vi "子界面-查看某框和报告生成.vi"(0 "框号":dbl format="%#_13g", 1 "框组":T4(array[cluster]), 2 "反射图":T1(plugin-control), 4 "标注图":T1(plugin-control)) -> ()   [LabVIEW 2018]
uses:
  <vilib>/vision/NI_Vision_Development_Module.lvlib
panel:
  in  "数据库UDL路径":path
  in  "写入数据库":bool
  out "ROI位置Y":i32
  out "ROI位置X":i32
  out "反射图ROI对应区域灰度表":u32[](graph)
  out "报告生成路径":path
  out "?":T1(plugin-control)
  out "Threshold Image":T1(plugin-control)
  in  "格式字符串 2":string="%f"
  in  "分隔符（'\\'代码显示）":string="\t"
  out "分层测量结果":dbl[][](array[numeric]) format="%.2f"
  out "分层类检测结果":string[][](table)
  out "Threshold Image":T1(plugin-control)
  out "Threshold Image":T1(plugin-control)
  out "缺陷分类的临界值":sgl
  out "反射图ROI的最大灰度值":sgl
  in  "返回 2":bool
  in  "报告生成":bool
  in  "反射法图像-面积阈值设置":T3(array[cluster]) {"Measurement Parameter" items=["Area"]; "下限" min=0 step=1; "上限" min=0 step=1}
  in  "穿透法图像-灰度阈值设置":cluster{"下限":dbl, "下限":dbl}(slide)={"下限"=0.0, "下限"=65.10638427734375} scale=0.0..255.0
  in  "保存结果":bool
  in  "部位":string
  in  "Color":u32[](array[colorbox])=[3381759, 16776770, 16777225, 6618880]
  in  "Overlay Type":u16[](array[ring])=[2, 1, 3, 0] items=["Rectangle", "Numbers", "Points", "Lines"]
  in  "Tab Control":T5
  out "穿透ROI":T1(plugin-control)
  out "Threshold Image":T1(plugin-control)
  out "?":T1(plugin-control)
  out "?":T1(plugin-control)
  out "Threshold Image":T1(plugin-control)
  out "Threshold Image":T1(plugin-control)
  out "弥散测量结果":dbl[][](array[numeric]) format="%.2f"
  in  "产品序号":string
  in  "测试人":string
  in  "分隔符（'\\'代码显示）":string="\t"
  in  "格式字符串":string="%f"
  out "弥散类检测结果":string[][](table)
  out "?":string
  out "面积 (pixels)":i32
  # "所选区域信息"
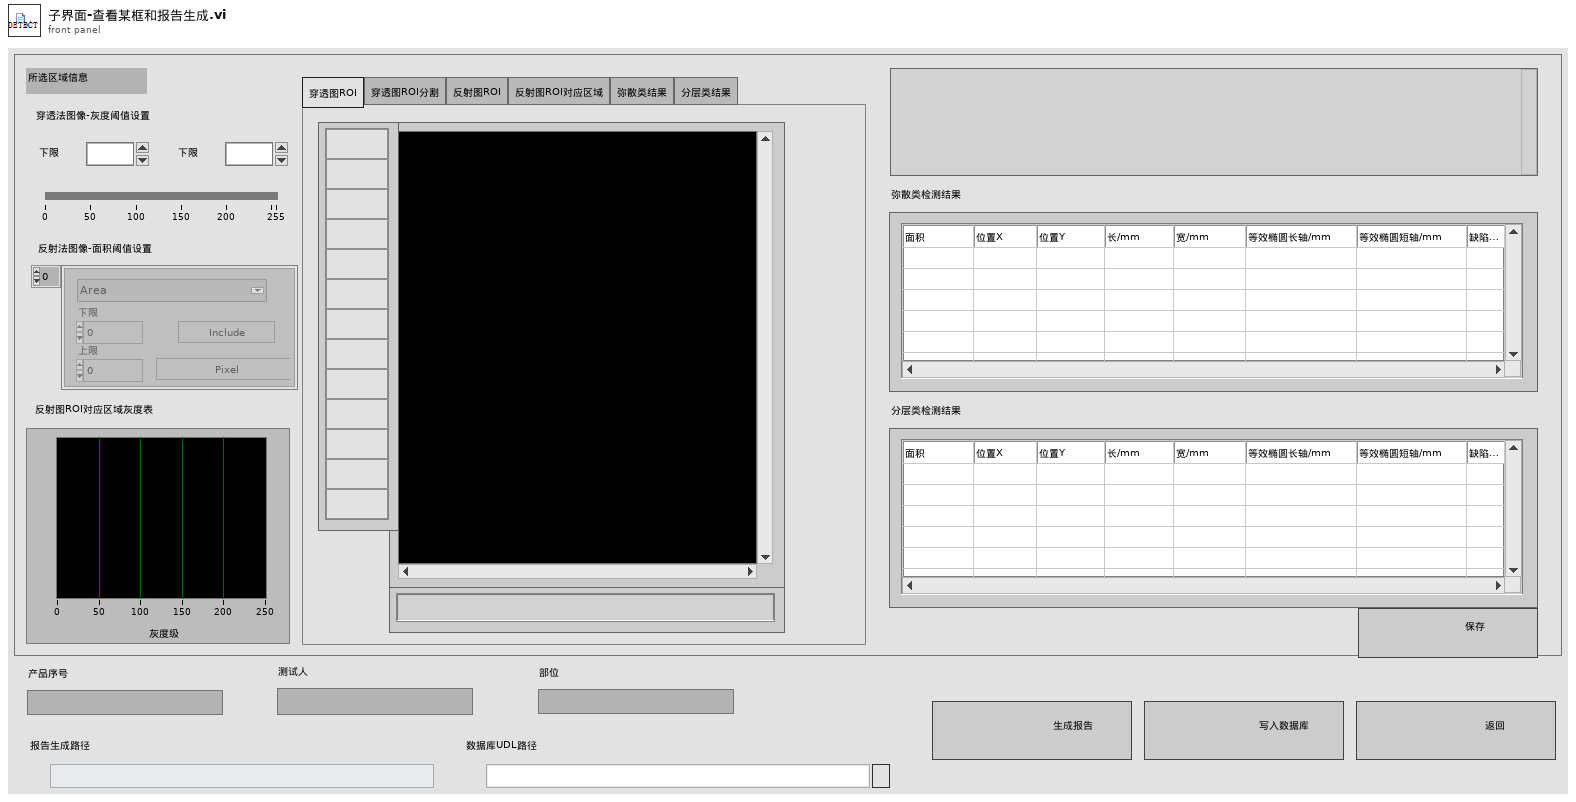
[diagram p1: front panel]
types:
  T1 = typedef "IMAQ Image.ctl" = refnum<image>
  T2 = typedef "Particle Parameters" = i32
  T3 = cluster{"Measurement Parameter":T2, "下限":i32, "上限":i32, "Range":bool, "Measurement Type":bool}[]
  T4 = cluster{"Global Rectangle":i32[], "Contours":cluster{"Contour Type":u32, "ROI Type":u32, "Points":i32[]}[]}[]
  T5 = typedef "控件 1.ctl" = enum32{"穿透图ROI", "穿透图ROI分割", "反射图ROI", "反射图ROI对应区域", "弥散类结果", "分层类结果"}
  T6 = typedef "Image Type" = u32
  T7 = cluster{"Global Rectangle":i32[], "Contours":cluster{"Contour Type":u32, "ROI Type":u32, "Points":i32[]}[]}
  T8 = cluster{"Pixel Measurements":T2[], "Overlay Type":u16[], "Color":u32[], "反射法图像-面积阈值设置":cluster{"Measurement Parameter":T2, "下限":i32, "上限":i32, "Range":bool, "Measurement Type":bool}[], "穿透法图像-灰度阈值设置":cluster{"下限":dbl, "下限":dbl}}
  T9 = cluster{"histogram":u32[], "Minimal Value":sgl, "Maximal Value":sgl, "Starting Value":sgl, "Interval Width":sgl, "Mean Value":sgl, "Standard  Variation":sgl, "Area (pixels)":i32}
  T10 = cluster{"Desired Font (Application)":enum16{"User-specified Font", "Application Font", "System Font", "Dialog Font"}, "[User-specified Font]":cluster{"Font Name":string, "Size":i16, "Strikeout?":bool, "Italic?":bool, "Underline?":bool, "Outline?":bool, "Shadow?":bool, "Bold?":bool, "Rotation Angle":dbl}, "Horizontal Alignment":i16, "Vertical Alignment":i16}
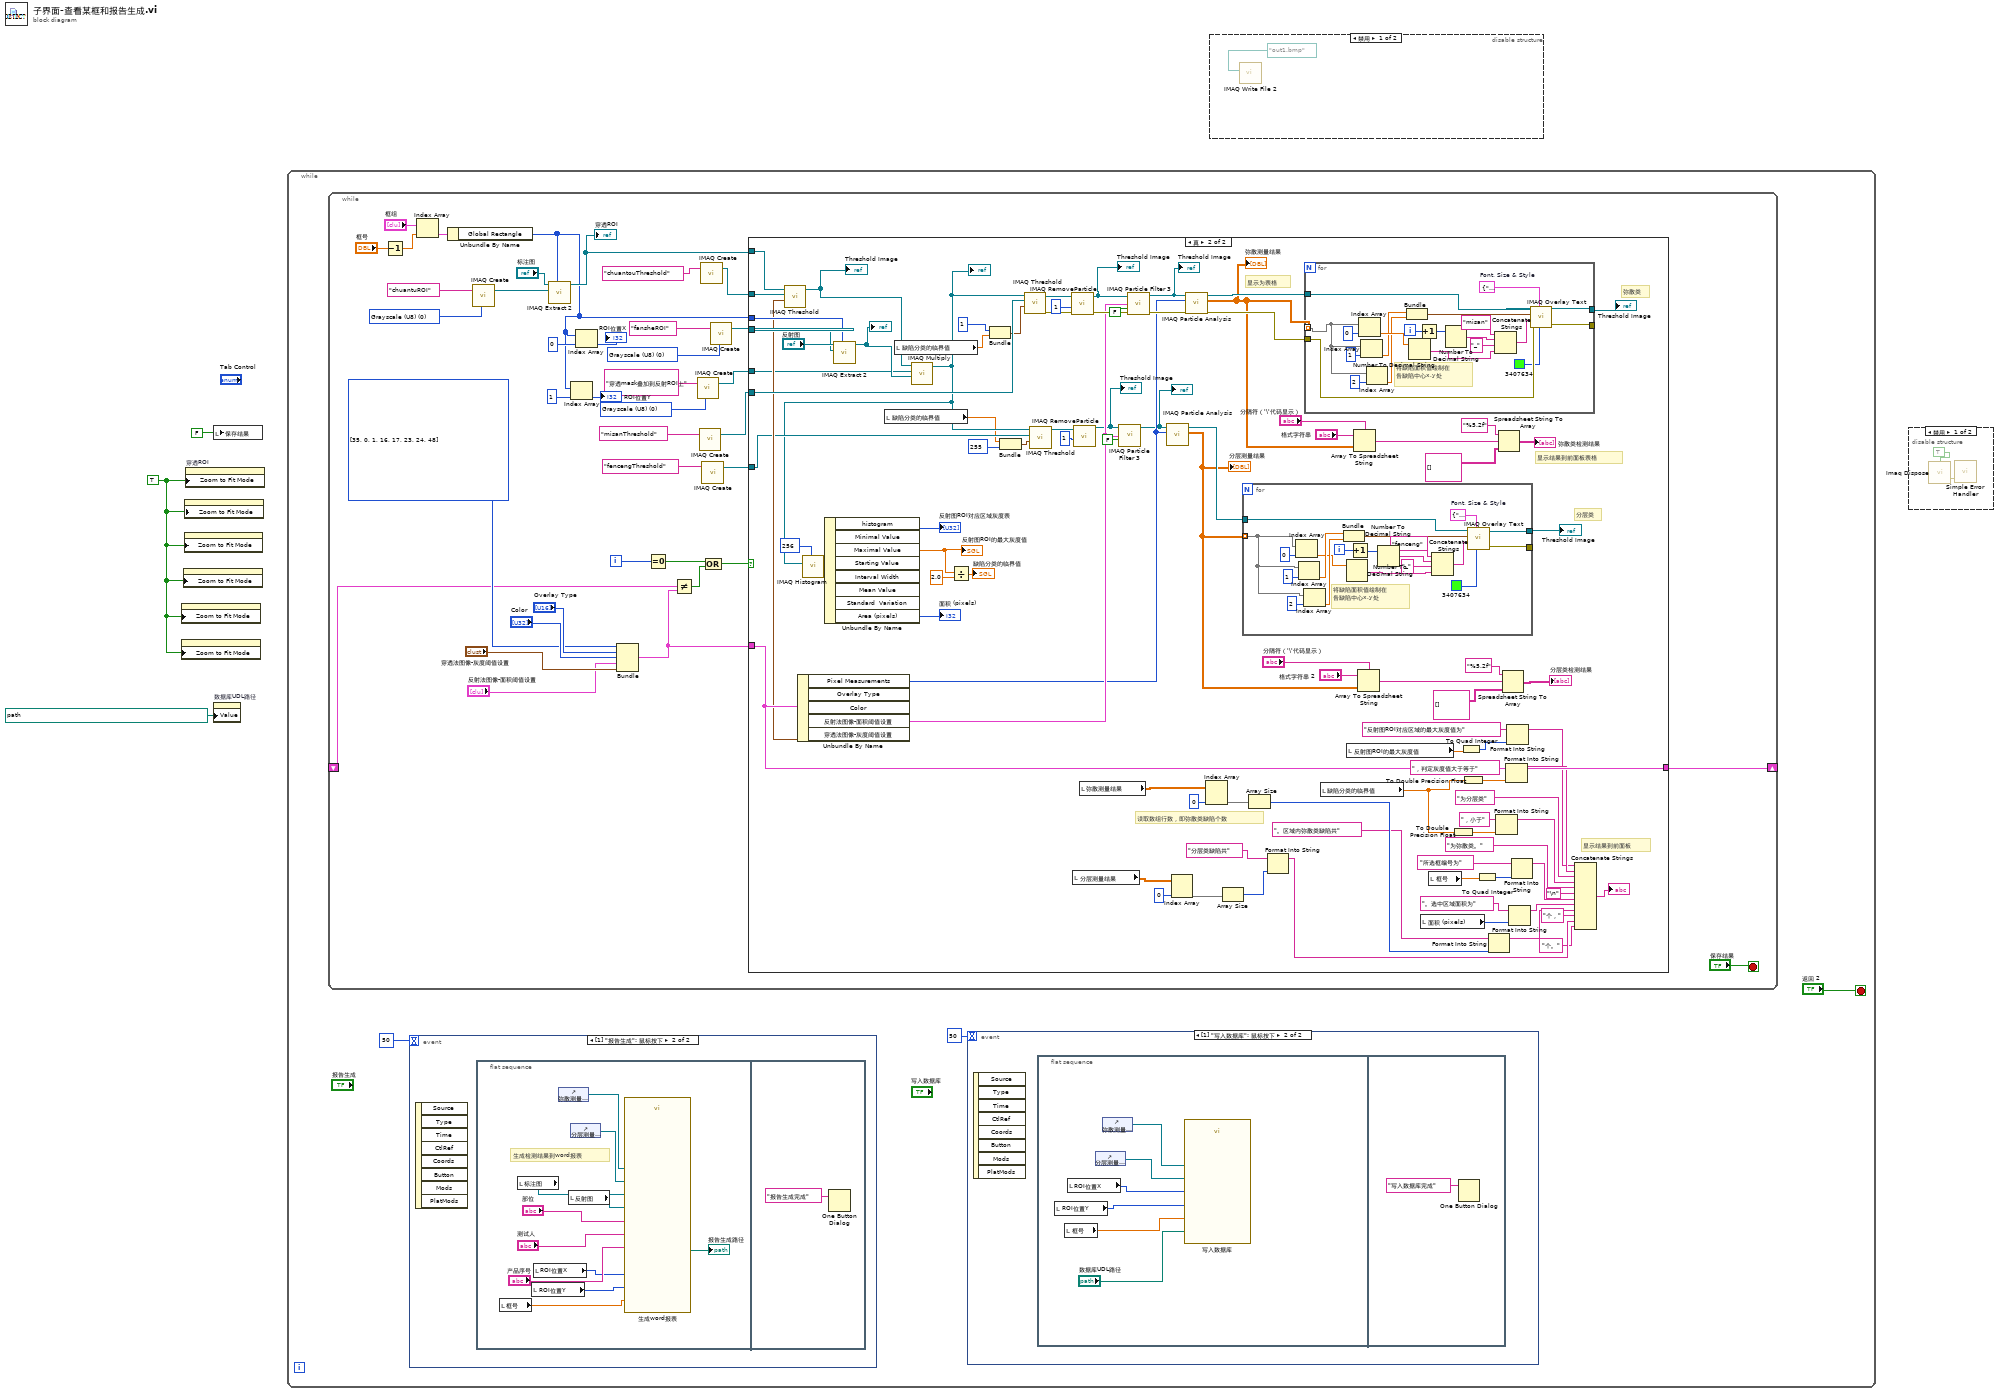
[diagram p0: block diagram]
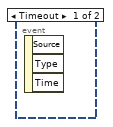
[diagram p3: hidden frame]
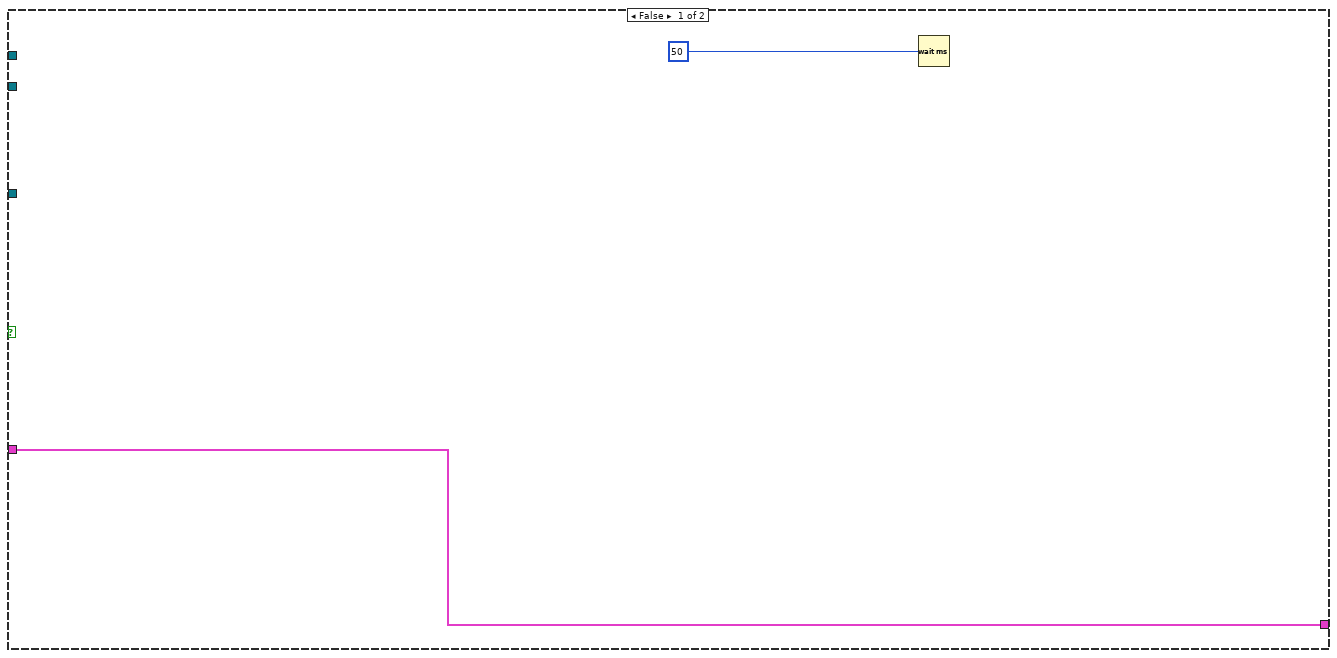
[diagram p4: hidden frame]
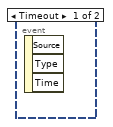
[diagram p5: hidden frame]
diagram:
  w2 = TRUE ("Zoom to Fit Mode")
  n1 = property class="ImageControl"("Zoom to Fit Mode"=w2) -> ()  [unwired: 2 in, 2 out]
  n2 = property class="ImageControl"("Zoom to Fit Mode"=w2) -> ()  [unwired: 2 in, 2 out]
  n3 = property class="ImageControl"("Zoom to Fit Mode"=w2) -> ()  [unwired: 2 in, 2 out]
  n4 = property class="ImageControl"("Zoom to Fit Mode"=w2) -> ()  [unwired: 2 in, 2 out]
  n5 = property class="ImageControl"("Zoom to Fit Mode"=w2) -> ()  [unwired: 2 in, 2 out]
  n6 = property on="穿透ROI" class="ImageControl"("Zoom to Fit Mode"=w2) -> ()  [unwired: 2 in, 2 out]
  n7 = local write "保存结果"(FALSE) -> ()
  n8 = property on="数据库UDL路径" class="Path"("Value"=path "E:/MyGithub/MyLabVIEW/晨光项目/代码/test.udl" ("数据库UDL路径")) -> ()  [unwired: 2 in, 2 out]
  n9 = while {
    stop <- "返回 2" stop-if-true
    n10 = while {
      shift-right: [w44] -> _
      shift-left: _ -> [w43]
      i -> [w48]
      stop <- "保存结果" stop-if-true
      w23 = T6 0 items=["Grayscale (U8)", "Grayscale (I16)", "Grayscale (SGL)", "Complex (CSG)", "RGB (U32)", "HSL (U32)", "RGB (U64)", "Grayscale (U16)"] ("Image Type")
      w29 = T6 0 items=["Grayscale (U8)", "Grayscale (I16)", "Grayscale (SGL)", "Complex (CSG)", "RGB (U32)", "HSL (U32)", "RGB (U64)", "Grayscale (U16)"] ("Image Type")
      w35 = T6 0 items=["Grayscale (U8)", "Grayscale (I16)", "Grayscale (SGL)", "Complex (CSG)", "RGB (U32)", "HSL (U32)", "RGB (U64)", "Grayscale (U16)"] ("Image Type")
      w50 = T2[] [35, 0, 1, 16, 17, 23, 24, 48] items=["Center of Mass X", "Center of Mass Y", "First Pixel X", "First Pixel Y", "Bounding Rect Left", "Bounding Rect Top", "Bounding Rect Right", "Bounding Rect Bottom", "Max Feret Diameter Start X", "Max Feret Diameter Start Y", "Max Feret Diameter End X", "Max Feret Diameter End Y", "Max Horiz. Segment Length Left", "Max Horiz. Segment Length Right", "Max Horiz. Segment Length Row", "-", "Bounding Rect Width", "Bounding Rect Height", "Bounding Rect Diagonal", "Perimeter", "Convex Hull Perimeter", "Holes' Perimeter", "Max Feret Diameter", "Equivalent Ellipse Major Axis", "Equivalent Ellipse Minor Axis", "Equivalent Ellipse Minor Axis (Feret)", "Equivalent Rect Long Side", "Equivalent Rect Short Side", "Equivalent Rect Diagonal", "Equivalent Rect Short Side (Feret)", "Average Horiz. Segment Length", "Average Vert. Segment Length", "Hydraulic Radius", "Waddel Disk Diameter", "-", "Area", "Holes' Area", "Particle & Holes' Area", "Convex Hull Area", "Image Area", "-", "Number of Holes", "Number of Horiz. Segments", "Number of Vert. Segments", "-", "Orientation", "Max Feret Diameter Orientation", "-", "% Area/Image Area", "% Area/(Particle & Holes' Area)", "Ratio of Equivalent Ellipse Axes", "Ratio of Equivalent Rect Sides", "-", "Elongation Factor", "Compactness Factor", "Heywood Circularity Factor", "Type Factor", "-", "Sum X", "Sum Y", "Sum XX", "Sum XY", "Sum YY", "Sum XXX", "Sum XXY", "Sum XYY", "Sum YYY", "-", "Moment of Inertia XX", "Moment of Inertia XY", "Moment of Inertia YY", "Moment of Inertia XXX", "Moment of Inertia XXY", "Moment of Inertia XYY", "Moment of Inertia YYY", "Norm. Moment of Inertia XX", "Norm. Moment of Inertia XY", "Norm. Moment of Inertia YY", "Norm. Moment of Inertia XXX", "Norm. Moment of Inertia XXY", "Norm. Moment of Inertia XYY", "Norm. Moment of Inertia YYY", "Hu Moment 1", "Hu Moment 2", "Hu Moment 3", "Hu Moment 4", "Hu Moment 5", "Hu Moment 6", "Hu Moment 7"] ("Pixel Measurements")
      n11 = Decrement(x="框号") -> (x-1=w37:dbl)
      n12 = Index Array(array="框组", index=w37) -> (element=w39:T7)
      n13 = Unbundle By Name(w39) -> ("Global Rectangle"=w15:i32[])
      n14 = call "IMAQ Create"("Image Name"="chuantuROI", "Image Type"=w35) -> ("New Image"=w38:T1)  [unwired: 3 in, 1 out]
      n15 = call "IMAQ Extract 2"("Optional Rectangle"=w15, "Image Dst"=w38, "Image Src"="标注图") -> ("Image Dst Out"=w26:T1)  [unwired: 7 in, 1 out]
      "穿透ROI" <- w26
      n16 = Index Array(array=w15, index=1 ("索引")) -> (element=→"ROI位置Y":i32)
      n17 = Index Array(array=w15, index=0 ("索引")) -> (element=→"ROI位置X":i32)
      n18 = Bundle("Pixel Measurements"=w50, "Overlay Type"="Overlay Type", "Color"="Color", "反射法图像-面积阈值设置"="反射法图像-面积阈值设置", "穿透法图像-灰度阈值设置"="穿透法图像-灰度阈值设置") -> (w27:T8)  [unwired: 1 in]
      n19 = Equal To 0?(x=w48) -> (x = 0?=w47:bool)
      n20 = Not Equal?(x=w43, y=w27) -> (x != y?=w46:bool)
      n21 = call "IMAQ Create"("Image Name"="穿透mask叠加到反射ROI上", "Image Type"=w23) -> ("New Image"=w22:T1)  [unwired: 3 in, 1 out]
      n22 = call "IMAQ Create"("Image Name"="misanThreshold") -> ("New Image"=w21:T1)  [unwired: 4 in, 1 out]
      n23 = call "IMAQ Create"("Image Name"="chuantouThreshold") -> ("New Image"=w31:T1)  [unwired: 4 in, 1 out]
      n24 = call "IMAQ Create"("Image Name"="fencengThreshold") -> ("New Image"=w19:T1)  [unwired: 4 in, 1 out]
      n25 = Compound Arithmetic op=OR(w47, w46) -> (w45:bool)
      n26 = call "IMAQ Create"("Image Name"="fansheROI", "Image Type"=w29) -> ("New Image"=w28:T1)  [unwired: 3 in, 1 out]
      n27 = case shown="真" w45 {
        tunnel: w27 -> [w53 w116]
        tunnel: [w53 w116] -> w44
        tunnel: w31 -> [_ w124]
        tunnel: w26 -> [_ w114]
        tunnel: w28 -> [_ w122]
        tunnel: w15 -> [_ w121]
        tunnel: w21 -> [_ w120]
        tunnel: w22 -> [_ w111]
        tunnel: w19 -> [_ w83]
        frame False {
          n28 = Wait (ms)(milliseconds to wait=u32 50) -> ()  [unwired: 1 out]
        }
        frame True {
          # "分层类"
          # "弥散类"
          # "显示结果到前面板"
          # "读取数组行数，即弥散类缺陷个数"
          # "显示结果到前面板表格"
          # "显示为表格"
          n29 = Unbundle By Name(w116) -> ("Pixel Measurements"=w74:T2[], "反射法图像-面积阈值设置"=w76:T3, "穿透法图像-灰度阈值设置"=w115:cluster{"下限":dbl, "下限":dbl})  [unwired: 2 out]
          n30 = call "IMAQ Threshold"("Range"=w115, "Image Dst"=w124, "Image Src"=w114) -> ("Image Dst Out"=w113:T1)  [unwired: 3 in, 5 out]
          "Threshold Image" <- w113
          n31 = call "IMAQ Extract 2"("Optional Rectangle"=w121, "Image Dst"=w122, "Image Src"="反射图") -> ("Image Dst Out"=w112:T1)  [unwired: 7 in, 1 out]
          "?" <- w112
          n32 = local read "缺陷分类的临界值"() -> (w79:sgl)
          n33 = local read "缺陷分类的临界值"() -> (w90:sgl)
          n34 = call "IMAQ Multiply"("Image Src A"=w113, "Image Dst"=w111, "Image Src B"=w112) -> ("Image Dst Out"=w82:T1)  [unwired: 4 in, 1 out]
          "?" <- w82
          n35 = call "IMAQ Histogram"("Number of Classes"=256, "Image"=w82) -> ("Histogram Report"=w119:T9)  [unwired: 8 in, 1 out]
          n36 = Unbundle By Name(w119) -> ("histogram"=→"反射图ROI对应区域灰度表":u32[], "Maximal Value"=w107:sgl, "Area (pixels)"=→"面积 (pixels)":i32)  [unwired: 5 out]
          "反射图ROI的最大灰度值" <- w107
          n37 = Divide(x=w107, y=sgl 2.0) -> (x/y=→"缺陷分类的临界值":sgl)
          n38 = Bundle(1, "缺陷分类的临界值"=w90) -> (w89:cluster{i32, "缺陷分类的临界值":sgl})  [unwired: 1 in]
          n39 = Bundle("缺陷分类的临界值"=w79, 255) -> (w81:cluster{"缺陷分类的临界值":sgl, i32})  [unwired: 1 in]
          n40 = call "IMAQ Threshold"("Range"=w89, "Image Dst"=w120, "Image Src"=w82) -> ("error out"=w148:errorcluster, "Image Dst Out"=w125:T1)  [unwired: 3 in, 4 out]
          n41 = call "IMAQ Threshold"("Range"=w81, "Image Dst"=w83, "Image Src"=w82) -> ("Image Dst Out"=w78:T1)  [unwired: 3 in, 5 out]
          n42 = call "IMAQ RemoveParticle"("error in (no error)"=w148, "Number of Erosion"=1, "Image Src"=w125) -> ("error out"=w147:errorcluster, "Image Dst Out"=w87:T1)  [unwired: 7 in]
          "Threshold Image" <- w87
          n43 = local read "分层测量结果"() -> (w62:dbl[][])
          n44 = call "IMAQ RemoveParticle"("Number of Erosion"=1, "Image Src"=w78) -> ("Image Dst Out"=w57:T1)  [unwired: 8 in, 1 out]
          "Threshold Image" <- w57
          n45 = local read "弥散测量结果"() -> (w84:dbl[][])
          n46 = call "IMAQ Particle Filter 3"("Image Src"=w57, "Selection Values"=w76, "Keep/Remove Particles (F)"=FALSE) -> ("Image Dst Out"=w56:T1)  [unwired: 10 in, 2 out]
          "?" <- w56
          n47 = call "IMAQ Particle Filter 3"("Image Src"=w87, "Selection Values"=w76, "Keep/Remove Particles (F)"=FALSE, "error in (no error)"=w147) -> ("Image Dst Out"=w86:T1, "error out"=w146:errorcluster)  [unwired: 9 in, 1 out]
          "Threshold Image" <- w86
          n48 = call "IMAQ Particle Analysis"("Pixel Measurements"=w74, "Image"=w56) -> ("Particle Measurements (Pixels)"=w68:dbl[][], "Image Out (duplicate)"=w73:T1)  [unwired: 4 in, 4 out]
          "分层测量结果" <- w68
          n49 = Index Array(array=w62, index (col)=0 ("禁用的索引 (列)")) -> (element=w64:dbl[])  [unwired: 1 in]
          n50 = call "IMAQ Particle Analysis"("error in (no error)"=w146, "Pixel Measurements"=w74, "Image"=w86) -> ("error out"=w144:errorcluster, "Particle Measurements (Pixels)"=w126:dbl[][], "Image Out (duplicate)"=w145:T1)  [unwired: 3 in, 3 out]
          "弥散测量结果" <- w126
          n51 = Index Array(array=w84, index (col)=0 ("禁用的索引 (列)")) -> (element=w132:dbl[])  [unwired: 1 in]
          n52 = Array Size(array=w64) -> (size(s)=w60:i32)
          n53 = for {
            tunnel: [w170] -> _
            tunnel: [w169] -> w72
            tunnel: w73 -> [w156]
            tunnel: w68 -> [w154] mode=indexing
            i -> [w151]
            w167 = T10 {"Desired Font (Application)"=enum."Application Font", "[User-specified Font]"={"Font Name"="", "Size"=12, "Strikeout?"=FALSE, "Italic?"=FALSE, "Underline?"=FALSE, "Outline?"=FALSE, "Shadow?"=FALSE, "Bold?"=FALSE, "Rotation Angle"=0.0}, "Horizontal Alignment"=0, "Vertical Alignment"=0}  # Font, Size & Style
            # "将缺陷面积值绘制在\n各缺陷中心x,y处"
            n54 = Index Array(array=w154, index=0 ("索引")) -> (element=w153:dbl)
            n55 = Index Array(array=w154, index=1 ("索引")) -> (element=w164:dbl)
            n56 = Index Array(array=w154, index=2 ("索引")) -> (element=w162:dbl)
            n57 = Bundle("Numeric"=w164, "Numeric"=w162) -> (w155:cluster{"Numeric":dbl, "Numeric":dbl})  [unwired: 1 in]
            n58 = Number To Decimal String(number=w153) -> (decimal integer string=w159:string)  [unwired: 1 in]
            n59 = Increment(x=w151) -> (x+1=w152:i32)
            n60 = Number To Decimal String(number=w152) -> (decimal integer string=w161:string)  [unwired: 1 in]
            n61 = Concatenate Strings("fenceng" ("字符串"), w161, "_", w159) -> (w158:string)
            n62 = call "IMAQ Overlay Text"("Text Color (black)"=u32 3407634, "Font, Size & Style"=w167, "String"=w158, "Origin"=w155, "Image"=w156) -> ("error out"=w170:errorcluster, "Image Out"=w169:T1)  [unwired: 5 in]
          }
          "Threshold Image" <- w72
          n63 = Array Size(array=w132) -> (size(s)=w134:i32)
          n64 = Format Into String(initial string="分层类缺陷共" ("初始字符串"), w60) -> (resulting string=w59:string)  [unwired: 2 in, 1 out]
          n65 = for {
            tunnel: w144 -> [w191]
            tunnel: [w190] -> _
            tunnel: [w189] -> w88
            tunnel: w145 -> [w187]
            tunnel: w126 -> [w180] mode=indexing
            i -> [w172]
            w186 = T10 {"Desired Font (Application)"=enum."Application Font", "[User-specified Font]"={"Font Name"="", "Size"=12, "Strikeout?"=FALSE, "Italic?"=FALSE, "Underline?"=FALSE, "Outline?"=FALSE, "Shadow?"=FALSE, "Bold?"=FALSE, "Rotation Angle"=0.0}, "Horizontal Alignment"=0, "Vertical Alignment"=0}  # Font, Size & Style
            # "将缺陷面积值绘制在\n各缺陷中心x,y处"
            n66 = Index Array(array=w180, index=0 ("索引")) -> (element=w185:dbl)
            n67 = Index Array(array=w180, index=1 ("索引")) -> (element=w182:dbl)
            n68 = Index Array(array=w180, index=2 ("索引")) -> (element=w179:dbl)
            n69 = Bundle("Numeric"=w182, "Numeric"=w179) -> (w178:cluster{"Numeric":dbl, "Numeric":dbl})  [unwired: 1 in]
            n70 = Number To Decimal String(number=w185) -> (decimal integer string=w175:string)  [unwired: 1 in]
            n71 = Increment(x=w172) -> (x+1=w171:i32)
            n72 = Number To Decimal String(number=w171) -> (decimal integer string=w177:string)  [unwired: 1 in]
            n73 = Concatenate Strings("misan" ("字符串"), w177, "_", w175) -> (w174:string)
            n74 = call "IMAQ Overlay Text"("Text Color (black)"=u32 3407634, "Font, Size & Style"=w186, "error in (no error)"=w191, "String"=w174, "Origin"=w178, "Image"=w187) -> ("error out"=w190:errorcluster, "Image Out"=w189:T1)  [unwired: 4 in]
          }
          "Threshold Image" <- w88
          n75 = local read "缺陷分类的临界值"() -> (w100:sgl)
          n76 = local read "反射图ROI的最大灰度值"() -> (w110:sgl)
          n77 = Array To Spreadsheet String(delimiter (Tab)="分隔符（'\\'代码显示）", array=w126, 3:"格式字符串") -> (spreadsheet string=w140:string)
          n78 = Array To Spreadsheet String(delimiter (Tab)="分隔符（'\\'代码显示）", array=w68, 3:"格式字符串 2") -> (spreadsheet string=w67:string)
          n79 = local read "面积 (pixels)"() -> (w131:i32)
          n80 = local read "框号"() -> (w136:dbl)
          n81 = To Double Precision Float(number=w100) -> (double precision float=w102:dbl)
          n82 = To Quad Integer(1:w110) -> (0:w109:i64)
          n83 = To Double Precision Float(number=w100) -> (double precision float=w104:dbl)
          n84 = To Quad Integer(1:w136) -> (0:w135:i64)
          n85 = Format Into String(initial string="。区域内弥散类缺陷共" ("初始字符串"), w134) -> (resulting string=w93:string)  [unwired: 2 in, 1 out]
          n86 = Format Into String(initial string="，小于" ("初始字符串"), w102) -> (resulting string=w98:string)  [unwired: 2 in, 1 out]
          n87 = Spreadsheet String To Array(format string="%5.2f", spreadsheet string=w140, array type (2D Dbl)=string[][] [] ("Array")) -> (array=→"弥散类检测结果":string[][])  [unwired: 1 in]
          n88 = Spreadsheet String To Array(format string="%5.2f", spreadsheet string=w67, array type (2D Dbl)=string[][] [] ("Array")) -> (array=→"分层类检测结果":string[][])  [unwired: 1 in]
          n89 = Format Into String(initial string="，判定灰度值大于等于" ("初始字符串"), w104) -> (resulting string=w96:string)  [unwired: 2 in, 1 out]
          n90 = Format Into String(initial string="反射图ROI对应区域的最大灰度值为" ("初始字符串"), w109) -> (resulting string=w95:string)  [unwired: 2 in, 1 out]
          n91 = Format Into String(initial string="。选中区域面积为" ("字符串"), w131) -> (resulting string=w94:string)  [unwired: 2 in, 1 out]
          n92 = Format Into String(initial string="所选框编号为" ("初始字符串"), w135) -> (resulting string=w137:string)  [unwired: 2 in, 1 out]
          n93 = Concatenate Strings(w95, w96, "为分层类" ("初始字符串"), w98, "为弥散类。" ("初始字符串"), "\n", w137, w94, w93, "个，" ("字符串"), w59, "个。" ("字符串")) -> (→"?":string)
        }
      }
    }
    n94 = event shown="[1] \"报告生成\": 鼠标按下" {
      selector: _ -> [_ _]
      dyn-events: _ -> [_ _]
      timeout: 50 -> [_ _]
      event Timeout {
        n95 = event-data() -> ()  [unwired: 1 in, 3 out]
      }
      event "报告生成": Mouse Down {
        n96 = event-data() -> ()  [unwired: 1 in, 8 out]
        n97 = flat-sequence {
          frame #0 {
            # "生成检测结果到word报表"
            n98 = local read "框号"() -> (w192:dbl)
            n99 = local read "标注图"() -> (w200:T1)
            n100 = local read "ROI位置Y"() -> (w193:i32)
            n101 = local read "ROI位置X"() -> (w194:i32)
            n102 = control-ref of="弥散测量结果"() -> (w198:refnum<vi>)
            n103 = local read "反射图"() -> (w201:T1)
            n104 = control-ref of="分层测量结果"() -> (w197:refnum<vi>)
            n105 = call "生成word报表.vi"("Array输入"=w198, "产品序号"="产品序号", "标注图"=w201, "Array输入 2"=w197, "测试人"="测试人", "部位"="部位", "ROI左上角X"=w194, "ROI左上角Y"=w193, "反射图"=w200, "框号"=w192) -> ("报告生成路径"=→"报告生成路径":path)  [unwired: 9 in]
          }
          frame #1 {
            n106 = One Button Dialog(message="报告生成完成" ("消息")) -> ()  [unwired: 1 in, 1 out]
          }
        }
      }
    }
    n107 = event shown="[1] \"写入数据库\": 鼠标按下" {
      selector: _ -> [_ _]
      dyn-events: _ -> [_ _]
      timeout: 50 -> [_ _]
      event Timeout {
        n108 = event-data() -> ()  [unwired: 1 in, 3 out]
      }
      event "写入数据库": Mouse Down {
        n109 = event-data() -> ()  [unwired: 1 in, 8 out]
        n110 = flat-sequence {
          frame #0 {
            n111 = local read "ROI位置Y"() -> (w8:i32)
            n112 = local read "框号"() -> (w7:dbl)
            n113 = local read "ROI位置X"() -> (w9:i32)
            n114 = control-ref of="分层测量结果"() -> (w10:refnum<vi>)
            n115 = control-ref of="弥散测量结果"() -> (w11:refnum<vi>)
            n116 = call "写入数据库.vi"("数据库UDL路径"="数据库UDL路径", "ROI左上角Y"=w8, "ROI左上角X"=w9, "框号"=w7, "Array输入 2"=w10, "Array输入"=w11) -> ()  [unwired: 6 in]
          }
          frame #1 {
            n117 = One Button Dialog(message="写入数据库完成" ("消息")) -> ()  [unwired: 1 in, 1 out]
          }
        }
      }
    }
  }
  n118 = disable-structure shown="禁用" {
    frame Disabled {
      n119 = call-poly "IMAQ Write File 2"("File Path"=path "out1.bmp") -> ()  [unwired: 9 in, 2 out]
    }
    frame Enabled {
    }
  }
  n120 = disable-structure shown="禁用" {
    frame Disabled {
      n121 = call "Imaq Dispose"("All Images? (No)"=TRUE) -> ("error out"=w206:errorcluster)  [unwired: 5 in]
      n122 = call <vilib>:"Simple Error Handler.vi"("error in (no error)"=w206) -> ()  [unwired: 4 in, 5 out]
    }
    frame Enabled {
    }
  }
